vi "Test.vi"   [LabVIEW 2016]
doc: "This VI starts when test mode begins, and will automatically be terminated when it ends. It will automatically publish I/O values, and you can add manual tests that can be invoked from the dashboard."
uses:
  <vilib>/Rock Robotics/Network Tables/NT Read String Array.vi
  <vilib>/Rock Robotics/Network Tables/NT Read Boolean.vi
types:
  T1 = typedef "WPI_EncoderDevRef.ctl" = cluster{"DevStatus":errorcluster, "EncoderIndex":T2, "CounterIndex":T3, "DistancePerCount":dbl, "Decoding Type":T4}
  T2 = typedef "FPGA_EncoderIdx.ctl" = enum8{"Enc 0", "Enc 1", "Enc 2", "Enc 3", "Enc 4", "Enc 5", "Enc 6", "Enc 7", "Invalid"}
  T3 = typedef "FPGA_CounterCtrSystemIndex.ctl" = enum8{"Ctr 0", "Ctr 1", "Ctr 2", "Ctr 3", "Ctr 4", "Ctr 5", "Ctr 6", "Ctr 7", "Invalid"}
  T4 = typedef "WPI_EncoderType.ctl" = enum16{"1x", "2x", "4x"}
  T5 = typedef "Command Status Info.ctl" = cluster{"Name":string, "Status":T6, "notifier out":T7}
  T6 = typedef "Completion Status.ctl" = enum16{"Successful", "Aborted", "Incomplete"}
  T7 = typedef "Completion Notifier.ctl" = refnum<notifier>
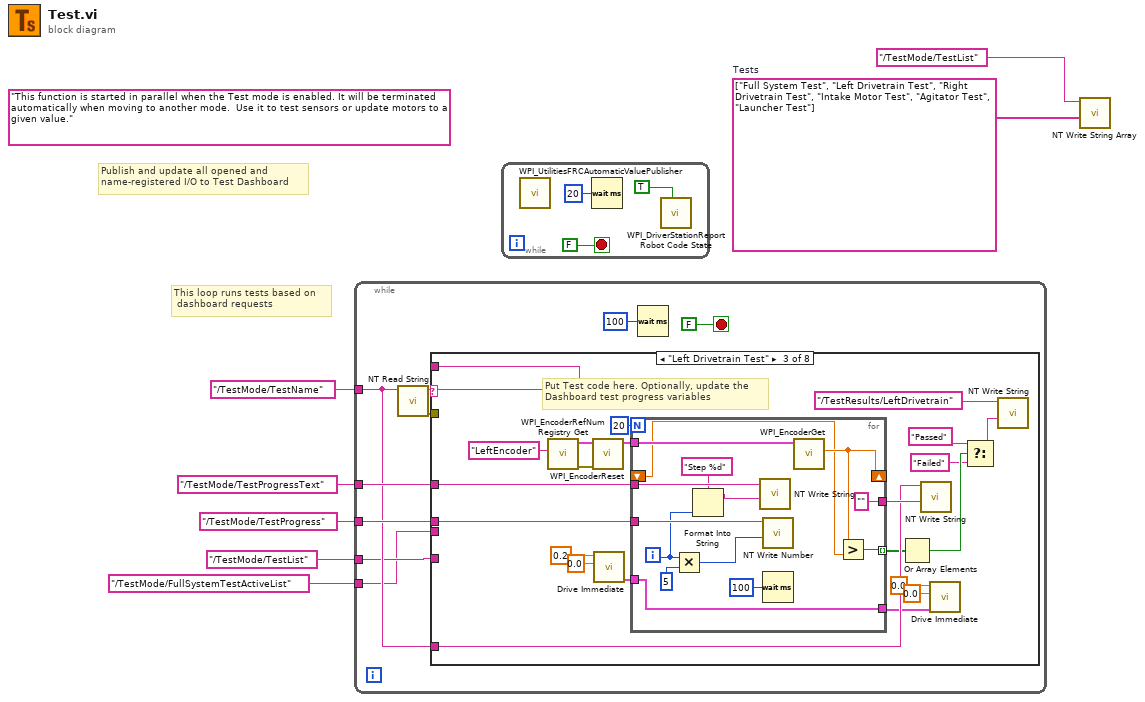
[diagram p0: block diagram]
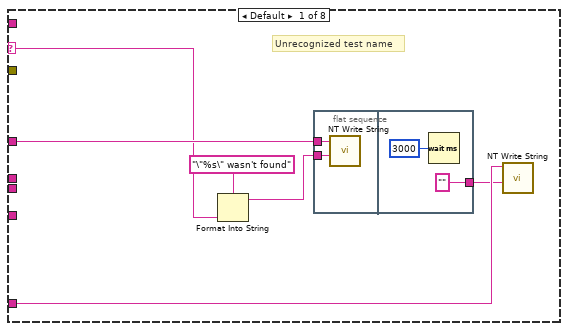
[diagram p2: hidden frame]
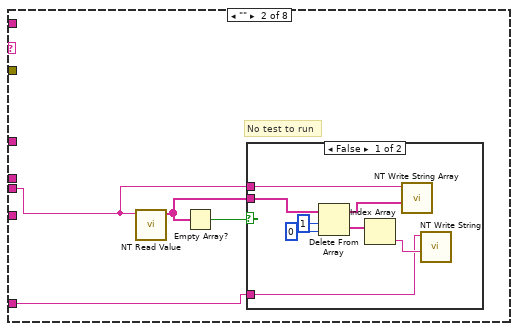
[diagram p3: hidden frame]
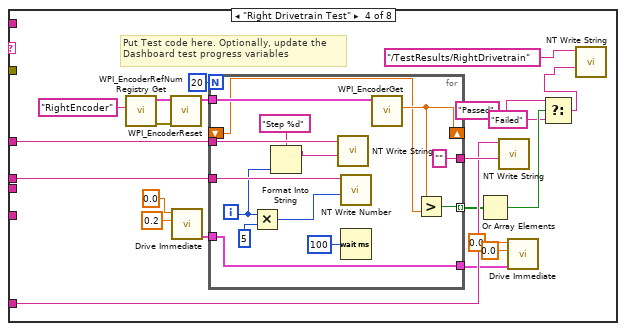
[diagram p5: hidden frame]
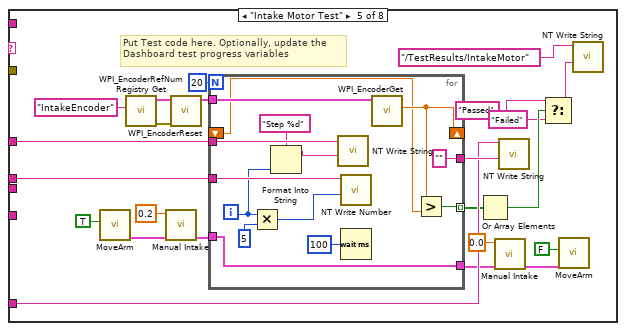
[diagram p6: hidden frame]
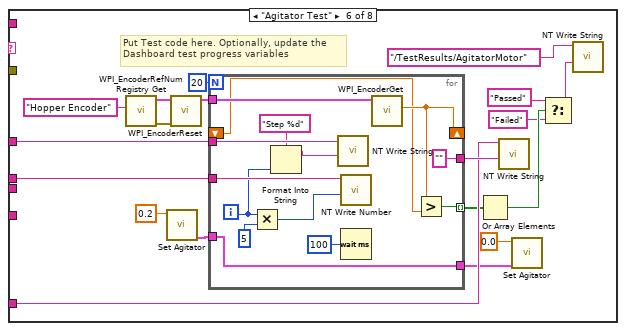
[diagram p7: hidden frame]
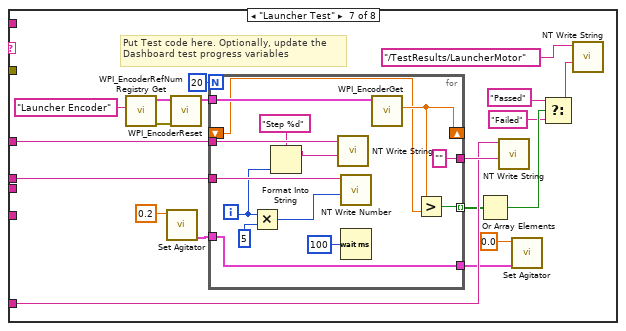
[diagram p8: hidden frame]
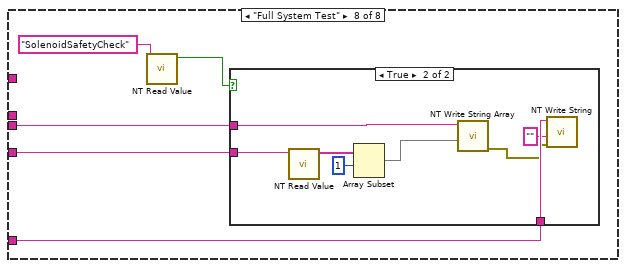
[diagram p9: hidden frame]
diagram:
  w4 = string[] ["Full System Test", "Left Drivetrain Test", "Right Drivetrain Test", "Intake Motor Test", "Agitator Test", "Launcher Test"]  # Tests
  (unwired) "This function is started in parallel when the Test mode is enabled. It will be terminated automatically when moving to another mode.  Use it to test sensors or update motors to a given value."
  # "This loop runs tests based on \n dashboard requests"
  # "Publish and update all opened and\nname-registered I/O to Test Dashboard"
  n1 = while {
    tunnel: "/TestMode/TestName" ("Name") -> [w11]
    tunnel: "/TestMode/TestProgressText" ("Name") -> [w14]
    tunnel: "/TestMode/TestProgress" ("Name") -> [w13]
    tunnel: "/TestMode/TestList" ("Name") -> [w9]
    tunnel: "/TestMode/FullSystemTestActiveList" ("Name") -> [w8]
    stop <- FALSE stop-if-true
    n2 = call <vilib>:"NT Read String.vi"("Name"=w11) -> ("error out"=w10:errorcluster, "String"=w12:string)  [unwired: 9 in]
    n3 = case shown="\"Left Drivetrain Test\"" w12 {
      selector: w12 -> [w21 _ _ _ _ _ _ _]
      tunnel: w11 -> [w18 w28 w56 w91 w128 w161 w194 w214]
      tunnel: w14 -> [w22 _ w44 w79 w122 w155 w188 _]
      tunnel: w13 -> [_ _ w59 w94 w131 w164 w197 _]
      tunnel: w12 -> [_ _ _ _ _ _ _ _]
      tunnel: w10 -> [_ _ _ _ _ _ _ _]
      tunnel: w9 -> [_ _ _ _ _ _ _ w216]
      tunnel: w8 -> [_ w27 _ _ _ _ _ w215]
      frame Default {
        # "Unrecognized test name"
        n4 = Format Into String(format string="\"%s\" wasn't found" ("Name"), w21) -> (resulting string=w20:string)  [unwired: 2 in, 1 out]
        n5 = flat-sequence {
          tunnel: w22 -> [w23]
          tunnel: w20 -> [w24]
          tunnel: ["" ("Name")] -> w17
          frame #0 {
            n6 = call <vilib>:"NT Write String.vi"("String"=w24, "Name"=w23) -> ()  [unwired: 9 in, 1 out]
          }
          frame #1 {
            n7 = Wait (ms)(milliseconds to wait=u32 3000) -> ()  [unwired: 1 out]
          }
        }
        n8 = call <vilib>:"NT Write String.vi"("String"=w17, "Name"=w18) -> ()  [unwired: 9 in, 1 out]
      }
      frame "" {
        # "No test to run"
        n9 = call-poly <vilib>:"NT Read Value.vi"("Name"=w27) -> ("String Array"=w29:string[])  [unwired: 9 in, 1 out]
        n10 = Empty Array?(array=w29) -> (empty?=w30:bool)
        n11 = case shown="False" w30 {
          tunnel: w29 -> [w38 _]
          tunnel: w28 -> [w33 _]
          tunnel: w27 -> [w32 _]
          frame False {
            n12 = Delete From Array(array=w38, length=1, index=0) -> (deleted portion=w35:string[], array with subset deleted=w31:string[])
            n13 = Index Array(array=w35) -> (element=w34:string)  [unwired: 1 in]
            n14 = call <vilib>:"NT Write String Array.vi"("String Array"=w31, "Name"=w32) -> ()  [unwired: 9 in, 1 out]
            n15 = call <vilib>:"NT Write String.vi"("String"=w34, "Name"=w33) -> ()  [unwired: 9 in, 1 out]
          }
          frame True {
          }
        }
      }
      frame "Left Drivetrain Test" {
        # "Put Test code here. Optionally, update the\nDashboard test progress variables"
        n16 = call <vilib>:"WPI_EncoderRefNum Registry Get.vi"("refnum name"="LeftEncoder") -> ("error out"=w50:errorcluster, "EncoderDevRef"=w51:T1)  [unwired: 9 in]
        n17 = call <vilib>:"WPI_EncoderReset.vi"("error in (no error)"=w50, "EncoderDevRef"=w51) -> ("EncoderDevRef"=w49:T1)  [unwired: 8 in, 1 out]
        n18 = call "Drive Immediate.vi"("Right Setpoint"=0.0, "Left Setpoint"=0.2) -> ("Command Info Out"=w53:T5)  [unwired: 9 in]
        n19 = for {
          N: 20 -> [_]
          tunnel: w59 -> [w73]
          tunnel: w44 -> [w71]
          tunnel: ["" ("String")] -> w57
          tunnel: w53 -> [w63]
          tunnel: w49 -> [w64]
          shift-right: [w62] -> _
          shift-left: _ -> [w61]
          tunnel: [w63] -> w46
          tunnel: [w60] -> w45 mode=indexing
          i -> [w68]
          n20 = Multiply(x=w68, y=u32 5 ("milliseconds to wait")) -> (x*y=w69:u32)
          n21 = Format Into String(format string="Step %d", w68) -> (resulting string=w66:string)  [unwired: 2 in, 1 out]
          n22 = call <vilib>:"NT Write String.vi"("String"=w66, "Name"=w71) -> ()  [unwired: 9 in, 1 out]
          n23 = call <vilib>:"NT Write Number.vi"("Numeric"=w69, "Name"=w73) -> ()  [unwired: 9 in, 1 out]
          n24 = Wait (ms)(milliseconds to wait=u32 100) -> ()  [unwired: 1 out]
          n25 = call <vilib>:"WPI_EncoderGet.vi"("EncoderDevRef"=w64) -> ("Distance"=w62:dbl)  [unwired: 5 in, 5 out]
          n26 = Greater?(x=w62, y=w61) -> (0:w60:bool)
        }
        n27 = Or Array Elements(Boolean array=w45) -> (logical OR=w43:bool)
        n28 = call <vilib>:"NT Write String.vi"("String"=w57, "Name"=w56) -> ()  [unwired: 9 in, 1 out]
        n29 = call "Drive Immediate.vi"("Command Info In"=w46, "Right Setpoint"=0.0, "Left Setpoint"=0.0) -> ()  [unwired: 8 in, 1 out]
        n30 = Select(t="Passed" ("String"), s=w43, f="Failed") -> (s? t:f=w39:string)
        n31 = call <vilib>:"NT Write String.vi"("String"=w39, "Name"="/TestResults/LeftDrivetrain") -> ()  [unwired: 9 in, 1 out]
      }
      frame "Right Drivetrain Test" {
        # "Put Test code here. Optionally, update the\nDashboard test progress variables"
        n32 = call <vilib>:"WPI_EncoderRefNum Registry Get.vi"("refnum name"="RightEncoder") -> ("error out"=w85:errorcluster, "EncoderDevRef"=w86:T1)  [unwired: 9 in]
        n33 = call <vilib>:"WPI_EncoderReset.vi"("error in (no error)"=w85, "EncoderDevRef"=w86) -> ("EncoderDevRef"=w84:T1)  [unwired: 8 in, 1 out]
        n34 = call "Drive Immediate.vi"("Right Setpoint"=0.2, "Left Setpoint"=0.0) -> ("Command Info Out"=w88:T5)  [unwired: 9 in]
        n35 = for {
          N: 20 -> [_]
          tunnel: w94 -> [w108]
          tunnel: w79 -> [w106]
          tunnel: ["" ("String")] -> w92
          tunnel: w88 -> [w98]
          tunnel: w84 -> [w99]
          shift-right: [w97] -> _
          shift-left: _ -> [w96]
          tunnel: [w98] -> w81
          tunnel: [w95] -> w80 mode=indexing
          i -> [w103]
          n36 = Multiply(x=w103, y=u32 5 ("milliseconds to wait")) -> (x*y=w104:u32)
          n37 = Format Into String(format string="Step %d", w103) -> (resulting string=w101:string)  [unwired: 2 in, 1 out]
          n38 = call <vilib>:"NT Write String.vi"("String"=w101, "Name"=w106) -> ()  [unwired: 9 in, 1 out]
          n39 = call <vilib>:"NT Write Number.vi"("Numeric"=w104, "Name"=w108) -> ()  [unwired: 9 in, 1 out]
          n40 = Wait (ms)(milliseconds to wait=u32 100) -> ()  [unwired: 1 out]
          n41 = call <vilib>:"WPI_EncoderGet.vi"("EncoderDevRef"=w99) -> ("Distance"=w97:dbl)  [unwired: 5 in, 5 out]
          n42 = Greater?(x=w97, y=w96) -> (0:w95:bool)
        }
        n43 = Or Array Elements(Boolean array=w80) -> (logical OR=w78:bool)
        n44 = call <vilib>:"NT Write String.vi"("String"=w92, "Name"=w91) -> ()  [unwired: 9 in, 1 out]
        n45 = call "Drive Immediate.vi"("Command Info In"=w81, "Right Setpoint"=0.0, "Left Setpoint"=0.0) -> ()  [unwired: 8 in, 1 out]
        n46 = Select(t="Passed" ("String"), s=w78, f="Failed") -> (s? t:f=w74:string)
        n47 = call <vilib>:"NT Write String.vi"("String"=w74, "Name"="/TestResults/RightDrivetrain") -> ()  [unwired: 9 in, 1 out]
      }
      frame "Intake Motor Test" {
        # "Put Test code here. Optionally, update the\nDashboard test progress variables"
        n48 = call "MoveArm.vi"("OnOff"=TRUE) -> ("Command Info Out"=w116:T5)  [unwired: 10 in]
        n49 = call <vilib>:"WPI_EncoderRefNum Registry Get.vi"("refnum name"="IntakeEncoder") -> ("error out"=w125:errorcluster, "EncoderDevRef"=w126:T1)  [unwired: 9 in]
        n50 = call "Manual Intake.vi"("Command Info In"=w116, "Setpoint"=0.2) -> ("Command Info Out"=w118:T5)  [unwired: 9 in]
        n51 = call <vilib>:"WPI_EncoderReset.vi"("error in (no error)"=w125, "EncoderDevRef"=w126) -> ("EncoderDevRef"=w124:T1)  [unwired: 8 in, 1 out]
        n52 = for {
          N: 20 -> [_]
          tunnel: w131 -> [w145]
          tunnel: w122 -> [w143]
          tunnel: ["" ("String")] -> w129
          tunnel: w118 -> [w135]
          tunnel: w124 -> [w136]
          shift-right: [w134] -> _
          shift-left: _ -> [w133]
          tunnel: [w135] -> w114
          tunnel: [w132] -> w123 mode=indexing
          i -> [w140]
          n53 = Multiply(x=w140, y=u32 5 ("milliseconds to wait")) -> (x*y=w141:u32)
          n54 = Format Into String(format string="Step %d", w140) -> (resulting string=w138:string)  [unwired: 2 in, 1 out]
          n55 = call <vilib>:"NT Write String.vi"("String"=w138, "Name"=w143) -> ()  [unwired: 9 in, 1 out]
          n56 = call <vilib>:"NT Write Number.vi"("Numeric"=w141, "Name"=w145) -> ()  [unwired: 9 in, 1 out]
          n57 = Wait (ms)(milliseconds to wait=u32 100) -> ()  [unwired: 1 out]
          n58 = call <vilib>:"WPI_EncoderGet.vi"("EncoderDevRef"=w136) -> ("Distance"=w134:dbl)  [unwired: 5 in, 5 out]
          n59 = Greater?(x=w134, y=w133) -> (0:w132:bool)
        }
        n60 = Or Array Elements(Boolean array=w123) -> (logical OR=w121:bool)
        n61 = call "Manual Intake.vi"("Command Info In"=w114, "Setpoint"=0.0 ("Left Setpoint")) -> ("Command Info Out"=w111:T5)  [unwired: 9 in]
        n62 = call <vilib>:"NT Write String.vi"("String"=w129, "Name"=w128) -> ()  [unwired: 9 in, 1 out]
        n63 = Select(t="Passed" ("String"), s=w121, f="Failed") -> (s? t:f=w109:string)
        n64 = call "MoveArm.vi"("Command Info In"=w111, "OnOff"=FALSE) -> ()  [unwired: 9 in, 1 out]
        n65 = call <vilib>:"NT Write String.vi"("String"=w109, "Name"="/TestResults/IntakeMotor") -> ()  [unwired: 9 in, 1 out]
      }
      frame "Agitator Test" {
        # "Put Test code here. Optionally, update the\nDashboard test progress variables"
        n66 = call <vilib>:"WPI_EncoderRefNum Registry Get.vi"("refnum name"="Hopper Encoder") -> ("error out"=w158:errorcluster, "EncoderDevRef"=w159:T1)  [unwired: 9 in]
        n67 = call "Set Agitator.vi"("Setpoint"=0.2) -> ("Command Info Out"=w148:T5)  [unwired: 10 in]
        n68 = call <vilib>:"WPI_EncoderReset.vi"("error in (no error)"=w158, "EncoderDevRef"=w159) -> ("EncoderDevRef"=w157:T1)  [unwired: 8 in, 1 out]
        n69 = for {
          N: 20 -> [_]
          tunnel: w164 -> [w178]
          tunnel: w155 -> [w176]
          tunnel: ["" ("String")] -> w162
          tunnel: w148 -> [w168]
          tunnel: w157 -> [w169]
          shift-right: [w167] -> _
          shift-left: _ -> [w166]
          tunnel: [w168] -> w147
          tunnel: [w165] -> w156 mode=indexing
          i -> [w173]
          n70 = Multiply(x=w173, y=u32 5 ("milliseconds to wait")) -> (x*y=w174:u32)
          n71 = Format Into String(format string="Step %d", w173) -> (resulting string=w171:string)  [unwired: 2 in, 1 out]
          n72 = call <vilib>:"NT Write String.vi"("String"=w171, "Name"=w176) -> ()  [unwired: 9 in, 1 out]
          n73 = call <vilib>:"NT Write Number.vi"("Numeric"=w174, "Name"=w178) -> ()  [unwired: 9 in, 1 out]
          n74 = Wait (ms)(milliseconds to wait=u32 100) -> ()  [unwired: 1 out]
          n75 = call <vilib>:"WPI_EncoderGet.vi"("EncoderDevRef"=w169) -> ("Distance"=w167:dbl)  [unwired: 5 in, 5 out]
          n76 = Greater?(x=w167, y=w166) -> (0:w165:bool)
        }
        n77 = Or Array Elements(Boolean array=w156) -> (logical OR=w154:bool)
        n78 = call <vilib>:"NT Write String.vi"("String"=w162, "Name"=w161) -> ()  [unwired: 9 in, 1 out]
        n79 = call "Set Agitator.vi"("Command Info In"=w147, "Setpoint"=0.0 ("Left Setpoint")) -> ()  [unwired: 9 in, 1 out]
        n80 = Select(t="Passed" ("String"), s=w154, f="Failed") -> (s? t:f=w150:string)
        n81 = call <vilib>:"NT Write String.vi"("String"=w150, "Name"="/TestResults/AgitatorMotor") -> ()  [unwired: 9 in, 1 out]
      }
      frame "Launcher Test" {
        # "Put Test code here. Optionally, update the\nDashboard test progress variables"
        n82 = call <vilib>:"WPI_EncoderRefNum Registry Get.vi"("refnum name"="Launcher Encoder") -> ("error out"=w191:errorcluster, "EncoderDevRef"=w192:T1)  [unwired: 9 in]
        n83 = call "Set Agitator.vi"("Setpoint"=0.2) -> ("Command Info Out"=w181:T5)  [unwired: 10 in]
        n84 = call <vilib>:"WPI_EncoderReset.vi"("error in (no error)"=w191, "EncoderDevRef"=w192) -> ("EncoderDevRef"=w190:T1)  [unwired: 8 in, 1 out]
        n85 = for {
          N: 20 -> [_]
          tunnel: w197 -> [w211]
          tunnel: w188 -> [w209]
          tunnel: ["" ("String")] -> w195
          tunnel: w181 -> [w201]
          tunnel: w190 -> [w202]
          shift-right: [w200] -> _
          shift-left: _ -> [w199]
          tunnel: [w201] -> w180
          tunnel: [w198] -> w189 mode=indexing
          i -> [w206]
          n86 = Multiply(x=w206, y=u32 5 ("milliseconds to wait")) -> (x*y=w207:u32)
          n87 = Format Into String(format string="Step %d", w206) -> (resulting string=w204:string)  [unwired: 2 in, 1 out]
          n88 = call <vilib>:"NT Write String.vi"("String"=w204, "Name"=w209) -> ()  [unwired: 9 in, 1 out]
          n89 = call <vilib>:"NT Write Number.vi"("Numeric"=w207, "Name"=w211) -> ()  [unwired: 9 in, 1 out]
          n90 = Wait (ms)(milliseconds to wait=u32 100) -> ()  [unwired: 1 out]
          n91 = call <vilib>:"WPI_EncoderGet.vi"("EncoderDevRef"=w202) -> ("Distance"=w200:dbl)  [unwired: 5 in, 5 out]
          n92 = Greater?(x=w200, y=w199) -> (0:w198:bool)
        }
        n93 = Or Array Elements(Boolean array=w189) -> (logical OR=w187:bool)
        n94 = call <vilib>:"NT Write String.vi"("String"=w195, "Name"=w194) -> ()  [unwired: 9 in, 1 out]
        n95 = call "Set Agitator.vi"("Command Info In"=w180, "Setpoint"=0.0 ("Left Setpoint")) -> ()  [unwired: 9 in, 1 out]
        n96 = Select(t="Passed" ("String"), s=w187, f="Failed") -> (s? t:f=w183:string)
        n97 = call <vilib>:"NT Write String.vi"("String"=w183, "Name"="/TestResults/LauncherMotor") -> ()  [unwired: 9 in, 1 out]
      }
      frame "Full System Test" {
        n98 = call-poly <vilib>:"NT Read Value.vi"("Name"="SolenoidSafetyCheck") -> ("Boolean"=w212:bool)  [unwired: 9 in, 1 out]
        n99 = case shown="True" w212 {
          tunnel: w216 -> [_ w224]
          tunnel: w215 -> [_ w220]
          tunnel: w214 -> [_ w219]
          frame False {
          }
          frame True {
            n100 = call-poly <vilib>:"NT Read Value.vi"("Name"=w224) -> ("String Array"=w223:string[])  [unwired: 9 in, 1 out]
            n101 = Array Subset(array=w223, index=1) -> (w221:string[])  [unwired: 1 in]
            n102 = call <vilib>:"NT Write String Array.vi"("String Array"=w221, "Name"=w220) -> ("error out"=w217:errorcluster)  [unwired: 9 in]
            n103 = call <vilib>:"NT Write String.vi"("error in"=w217, "String"="", "Name"=w219) -> ()  [unwired: 8 in, 1 out]
          }
        }
      }
    }
    n104 = Wait (ms)(milliseconds to wait=u32 100) -> ()  [unwired: 1 out]
  }
  n105 = while {
    stop <- FALSE stop-if-true
    n106 = call <vilib>:"WPI_UtilitiesFRCAutomaticValuePublisher.vi"() -> ()  [unwired: 12 in]
    n107 = Wait (ms)(milliseconds to wait=u32 20) -> ()  [unwired: 1 out]
    n108 = call <vilib>:"WPI_DriverStationReport Robot Code State.vi"("Test"=TRUE ("Autonomous")) -> ()  [unwired: 10 in, 1 out]
  }
  n109 = call <vilib>:"NT Write String Array.vi"("String Array"=w4, "Name"="/TestMode/TestList") -> ()  [unwired: 9 in, 1 out]
